vi "CameraInit.vi"() -> (0 "error out":errorcluster)   [LabVIEW 2018]
uses:
  VsyCam.dll
panel:
  out "增益":dbl
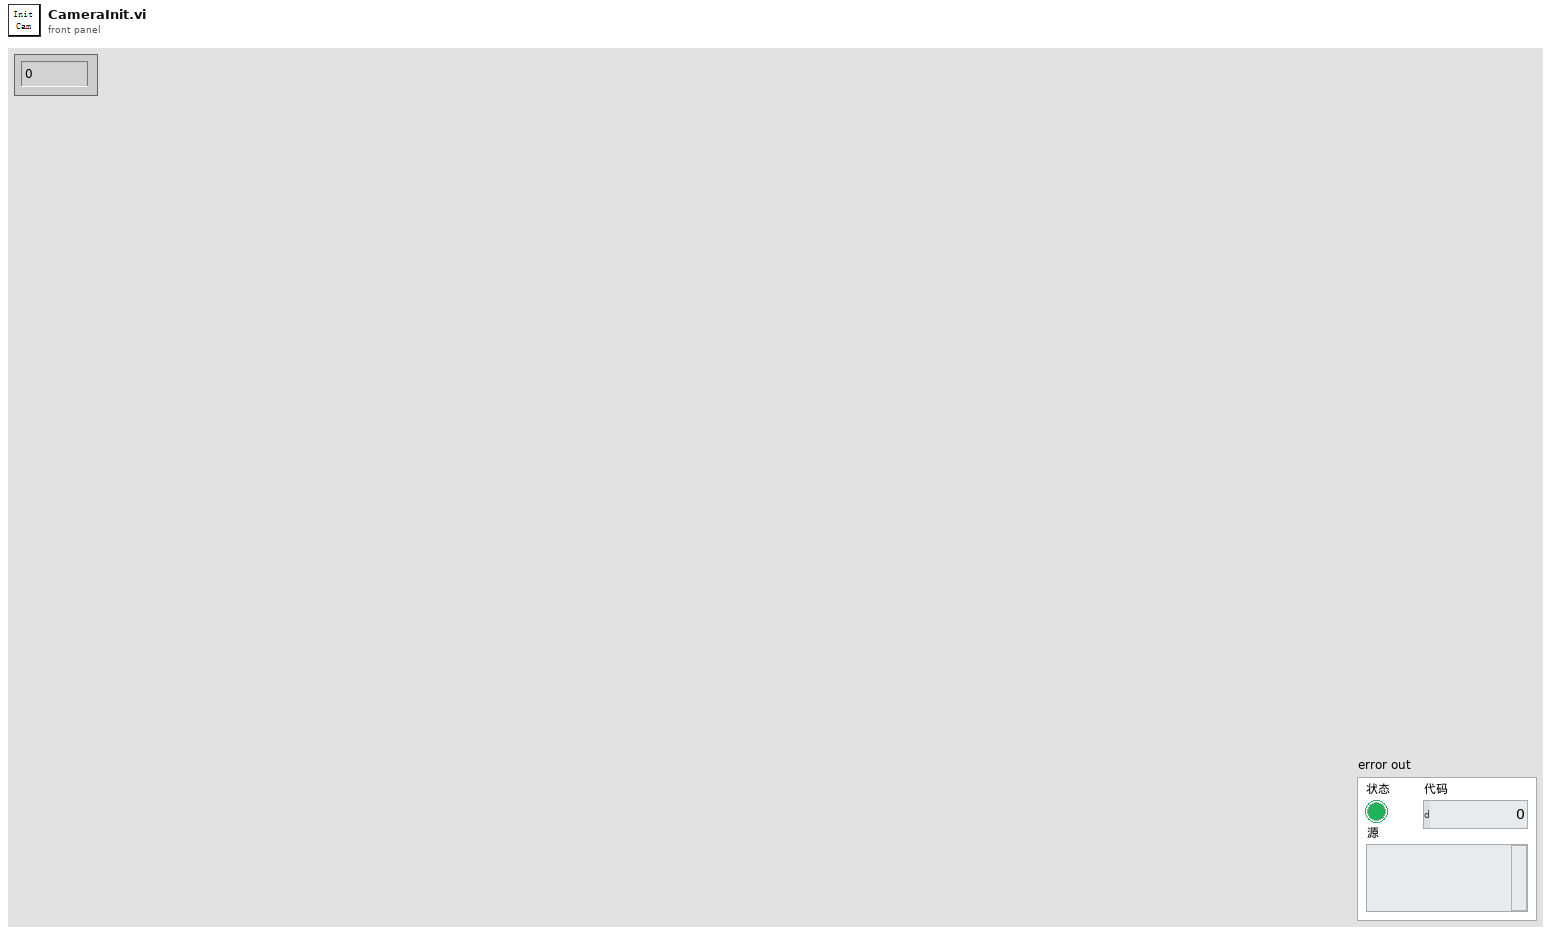
[diagram p1: front panel]
types:
  T1 = typedef "IMAQ Image.ctl" = refnum<image>
  T2 = cluster{"示波器":cluster{"Channel (0:Channel 1)":enum16{"Channel 1", "Channel 2", "Channel 3", "Channel 4"}, "电压范围":dbl, "触发电压":dbl, "时间范围":dbl, " 示波器VISA":refnum<visa-resource-name>, "时间范围 标签":u64, "电压范围 标签":u64, "触发电压 标签":u64}, "光谱仪":cluster{"Channel (0:Channel 1)":enum16{"Channel 1", "Channel 2", "Channel 3", "Channel 4"}, "电压范围":u64, "触发电压":u64, "时间范围":u64}, " 近场相机":cluster{"曝光时间":dbl, "模拟增益":i32, "控制套接字":i32, "IP 地址":string, " 采集套接字":i32, "  版本号":i32, "ImageData":T1, "  增益最大":i32, "  增益最小":i32, " 曝光最大":i32, " 曝光最小":i32, " 帧速":i32, " 同步切换":i32, "  曝光缩放":i32}, " 偏振仪":cluster{"电压范围":u64, "触发电压":u64, "时间范围":u64, "波长范围":enum16{"可见光 400-700nm", "近红外 700-1100nm"}, "可见光偏振测量仪VISA":refnum<visa-resource-name>, "近红外偏振测量仪VISA":refnum<visa-resource-name>}, " 功率计":cluster{"通道":enum16{"Channel 1", "Channel 2"}, "工作波长":u32, "单位":u64, "时间范围":u64, "IP地址":string, "端口":u32}, "能量计":cluster{"通道":enum16{"Channel 1", "Channel 2"}, "工作波长":u32, "单位":u64, "时间范围":u64, "IP地址":string, "端口":u32, "能量计量程":enum16{"200uJ", "20uJ", "2uJ", "200nJ"}}, "电机":cluster{"Channel (0:Channel 1)":enum16{"Channel 1", "Channel 2", "Channel 3", "Channel 4"}, "电压范围":u64, "触发电压":u64, "时间范围":u64}, " 远场相机":cluster{"曝光时间":i32, "模拟增益":i32, "控制套接字":i32, "IP 地址":string, " 采集套接字":i32, "  版本号":i32, "ImageData":T1, "  增益最大":i32, "  增益最小":i32, " 曝光最大":i32, " 曝光最小":i32, " 帧速":i32, " 同步切换":i32, "  曝光缩放":i32}}
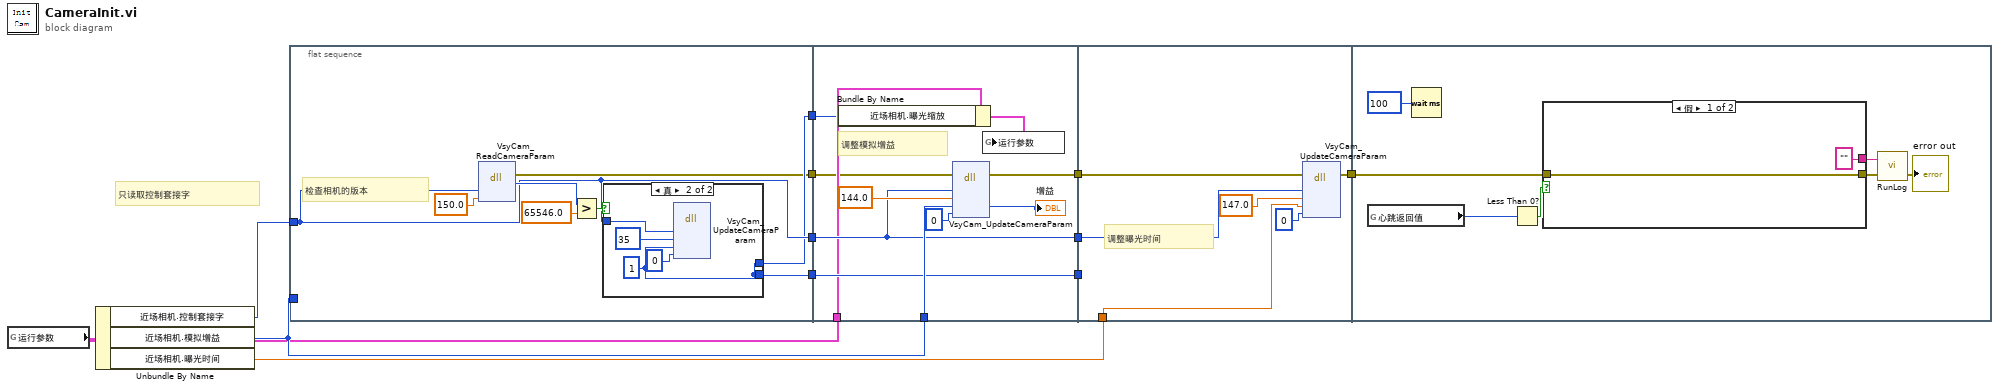
[diagram p0: block diagram]
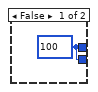
[diagram p2: hidden frame]
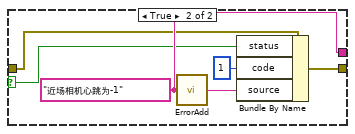
[diagram p3: hidden frame]
diagram:
  # "只读取控制套接字"
  n1 = global read "参数.vi" "运行参数"() -> (w5:T2)
  n2 = Unbundle By Name(w5) -> ("近场相机.控制套接字"=w12:i32, "近场相机.模拟增益"=w9:i32, "近场相机.曝光时间"=w11:dbl)
  n3 = flat-sequence {
    tunnel: w9 -> [_]
    tunnel: w12 -> [w16]
    tunnel: [w16] -> w10
    tunnel: [w15] -> w6
    tunnel: [w14] -> w4
    tunnel: [w13] -> w3
    tunnel: w10 -> [w32]
    tunnel: w9 -> [w33]
    tunnel: [w32] -> w8
    tunnel: [w31] -> w7
    tunnel: w6 -> [w31]
    tunnel: w5 -> [w30]
    tunnel: w4 -> [w29]
    tunnel: w3 -> [w28]
    tunnel: [w27] -> w2
    tunnel: w11 -> [w37]
    tunnel: w8 -> [w40]
    tunnel: w7 -> [_]
    tunnel: w2 -> [w39]
    tunnel: [w38] -> w1
    tunnel: w1 -> [w44]
    frame #0 {
      # "检查相机的版本"
      n4 = dll-call lib="PTH2?abs D做的项目航天测量软件相机\nVsyCam.dll" fn="VsyCam_ReadCameraParam"("sockFd"=w16, "cmd"=150.0) -> (error out=w13:errorcluster, "返回类型"=w18:i32)  [unwired: 5 in, 1 out]
      n5 = Greater?(x=w18, y=65546.0) -> (0:w17:bool)
      n6 = case shown="真" w17 {
        tunnel: [w21 w22] -> w15
        tunnel: w16 -> [_ w23]
        tunnel: [w21 w22] -> w14
        frame False {
          w21 = 100
        }
        frame True {
          w22 = 1
          n7 = dll-call lib="PTH2?abs D做的项目航天测量软件相机\nVsyCam.dll" fn="VsyCam_UpdateCameraParam"("sockFd"=w23, "command"=35, "value"=w22, "ack"=0) -> ()  [unwired: 8 in, 2 out]
        }
      }
    }
    frame #1 {
      # "调整模拟增益"
      n8 = Bundle By Name(cluster=w30, "近场相机.曝光缩放"=w29) -> (w26:T2)
      n9 = dll-call lib="PTH2?abs D做的项目航天测量软件相机\nVsyCam.dll" fn="VsyCam_UpdateCameraParam"(error in=w28, "sockFd"=w32, "command"=144.0, "value"=w33, "ack"=0) -> (error out=w27:errorcluster, "value"=→"增益":i32)  [unwired: 6 in, 1 out]
      n10 = global write "参数.vi" "运行参数"(w26) -> ()
    }
    frame #2 {
      # "调整曝光时间"
      n11 = dll-call lib="PTH2?abs D做的项目航天测量软件相机\nVsyCam.dll" fn="VsyCam_UpdateCameraParam"(error in=w39, "sockFd"=w40, "command"=147.0, "value"=w37, "ack"=0) -> (error out=w38:errorcluster)  [unwired: 7 in, 1 out]
    }
    frame #3 {
      n12 = global read "globalMessage.vi" "心跳返回值"() -> (w46:i32)
      n13 = Wait (ms)(milliseconds to wait=u32 100 ("等待时间（毫秒）")) -> ()  [unwired: 1 out]
      n14 = Less Than 0?(x=w46) -> (x < 0?=w45:bool)
      n15 = case shown="假" w45 {
        selector: w45 -> [_ w54]
        tunnel: ["" w57] -> w48
        tunnel: w44 -> [w51 w53]
        tunnel: [w51 w52] -> w43
        frame False {
        }
        frame True {
          w57 = "近场相机心跳为-1" ("source")
          n16 = call "ErrorAdd.vi"("source"=w57) -> ("Errorout Souce"=w55:string)
          n17 = Bundle By Name(cluster=w53, "status"=w54, "code"=1, "source"=w55) -> (w52:errorcluster)
        }
      }
      n18 = call "RunLog.vi"("error in"=w43, "Message"=w48) -> ("error out"=→"error out":errorcluster)  [unwired: 1 in]
    }
  }
